vi "SimpleExample.vi"(0 "End Session":bool, 2 "Properties in Service":string[](array[string])=["Button", "Potentiometer", "Temperature", "Photocell", "Button2"]) -> (1 "Properties from ThingWorx":string[][](array[string])=[["Button", "true"], ["Button2", "true"], ["description", ""], ["isConnected", "false"], ["lastConnection", "1970-01-01T00:00:00.000Z"], ["name", "GenericEdge"], ["Photocell", "200.0"], ["Potentiometer", "234.0"], ["tags", "GenericRemoteEdge:Example"], ["Temperature", "0.242"], ["thingTemplate", "GenericThingTemplate"]])   [LabVIEW 2015]
uses:
  <vilib>/httpClient/LabVIEWHTTPClient.lvlib
panel:
  in  "Property Values":string[][](array[string])=[["Button", "1"], ["Potentiometer", "90"], ["Temperature", "25"], ["Photocell", "75"], ["Button2", "0"]]
  in  "Input Array":string[](array[string])=["52.202.159.58", "80", "GenericThing", "0aae8b5f-871a-4973-bdf2-199fabb27dcb", "UpdateValues"]
  out "error out":errorcluster
  # "Before running program, input values for \"Thing Name,\" \"App Key,\" \"ThingWorx Server Address,\" \"Port,\"Service Name,\" and \"Properties in Service.\"\nTo change the values of all properties at once, click continuous. If you would like to change individual property values, unclick the continuous\nbutton and select the property you would like to change in the dropdown menu and enter your desired value."
  # "Input Array:\n0. ThingWorx Server Address\n1. Port\n2. Thing Name\n3. App Key\n4. Service Name"
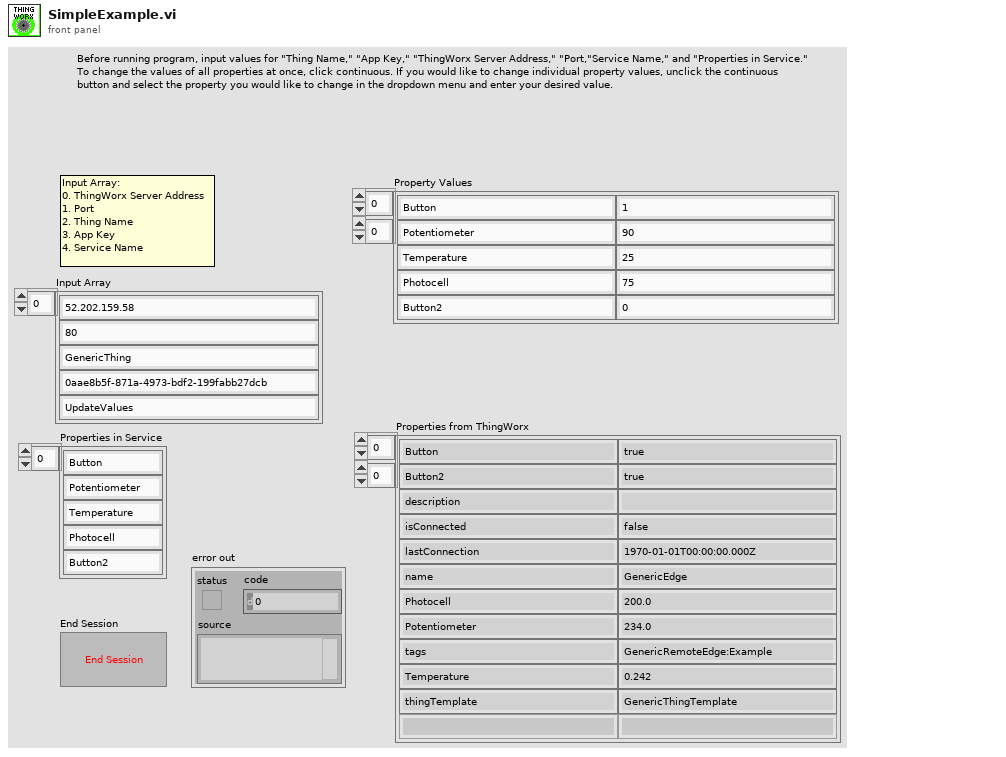
[diagram p1: front panel]
types:
  T1 = typedef "LabVIEWHTTPClient.lvlib/ClientHandle.ctl" = refnum<k1>
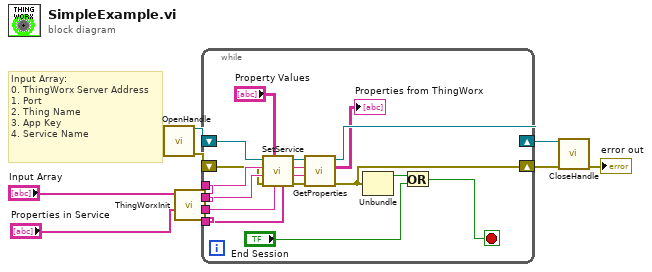
[diagram p0: block diagram]
diagram:
  # "Input Array:\n0. ThingWorx Server Address\n1. Port\n2. Thing Name\n3. App Key\n4. Service Name"
  n1 = call <vilib>:"OpenHandle.vi"() -> ("client handle out"=w6:T1, "error out"=w5:errorcluster)  [unwired: 14 in]
  n2 = call "ThingWorxInit.vi"("Properties"="Properties in Service", "Input Array"="Input Array") -> ("Properties Out"=w1:string[], "Service Name"=w3:string, "appKey"=w10:string, "url beginning"=w11:string)  [unwired: 6 in]
  n3 = while {
    tunnel: w11 -> [w24]
    shift-right: [w28] -> w8
    shift-left: w6 -> [w23]
    shift-right: [w15] -> w9
    shift-left: w5 -> [w14]
    tunnel: w10 -> [w22]
    tunnel: w3 -> [w17]
    tunnel: w1 -> [w13]
    stop <- w27 stop-if-true
    n4 = call "SetService.vi"("Properties in Service"=w13, "Service Name"=w17, "Properties"="Property Values", "error in"=w14, "appKey"=w22, "uri beginning"=w24, "client handle"=w23) -> ("error out"=w16:errorcluster, "appKey out"=w19:string, "uri beginning out"=w18:string, "client handle out"=w20:T1)  [unwired: 1 out]
    n5 = call "GetProperties.vi"("error in (no error)"=w16, "appKey"=w19, "url beginning"=w18, "client handle"=w20) -> ("error out"=w15:errorcluster, "Array"=→"Properties from ThingWorx":string[][], "client handle out"=w28:T1)  [unwired: 3 in, 2 out]
    n6 = Unbundle(w15) -> ("status"=w25:bool)  [unwired: 2 out]
    n7 = Or(x=w25, y="End Session") -> (x .or. y?=w27:bool)
  }
  n8 = call <vilib>:"CloseHandle.vi"("client handle"=w8, "error in (no error)"=w9) -> ("error out"=→"error out":errorcluster)  [unwired: 13 in]
